vi "case1_selector.vi"(0 "T1":dbl, 2 "T2":dbl, 3 "Delay":dbl) -> (6 "overlap select":T1(ring))   [LabVIEW 2015]
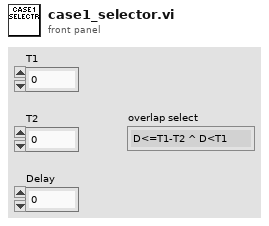
[diagram p1: front panel]
types:
  T1 = enum16{"D<=T1-T2 ^ D<T1", "D<T1 ^ D>T1-T2", "D>=T1"}
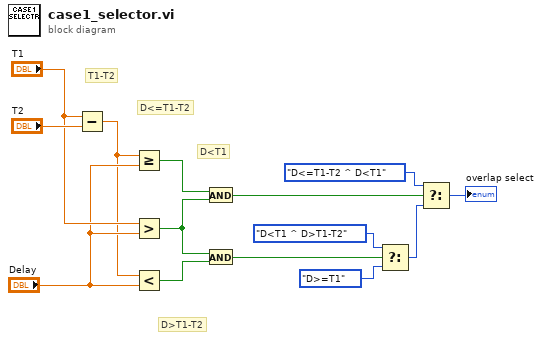
[diagram p0: block diagram]
diagram:
  # "D>T1-T2"
  # "D<=T1-T2"
  # "T1-T2"
  # "D<T1"
  n1 = Subtract(x="T1", y="T2") -> (x-y=w2:dbl)
  n2 = Greater Or Equal?(x=w2, y="Delay") -> (x >= y?=w8:bool)
  n3 = Greater?(x="T1", y="Delay") -> (0:w4:bool)
  n4 = Less?(x=w2, y="Delay") -> (x < y?=w5:bool)
  n5 = And(x=w8, y=w4) -> (x .and. y?=w7:bool)
  n6 = And(x=w4, y=w5) -> (x .and. y?=w6:bool)
  n7 = Select(t=T1."D<T1 ^ D>T1-T2", s=w6, f=T1."D>=T1") -> (s? t:f=w14:T1)
  n8 = Select(t=T1."D<=T1-T2 ^ D<T1", s=w7, f=w14) -> (s? t:f=→"overlap select":T1)
